vi "Intake_Hopper_Pneumatic_Safety_Interlocks.vi"(5 "extend delay(ms)":u32=1000, 7 "retract delay(ms)":u32=1000, 9 "Hopper Input":T1=enum."Reverse", 10 "Intake Input":T1=enum."Reverse") -> (1 "Hopper Output":T1=enum."Reverse", 2 "Intake Output":T1=enum."Reverse")   [LabVIEW 2019]
uses:
  <vilib>/Rock Robotics/WPI/Solenoid/WPI_SolenoidValue.ctl
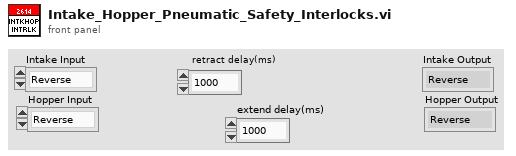
[diagram p1: front panel]
types:
  T1 = typedef "WPI_SolenoidValue.ctl" = enum16{"Off", "On", "Forward", "Reverse"}
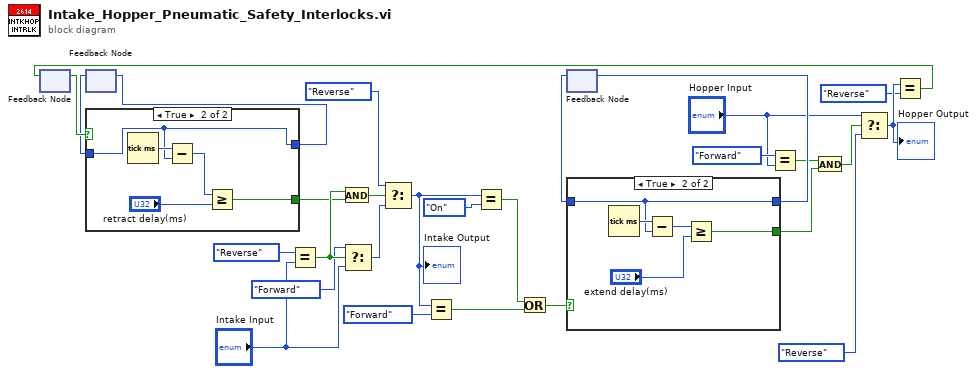
[diagram p0: block diagram]
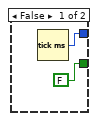
[diagram p2: hidden frame]
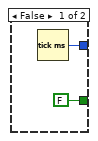
[diagram p3: hidden frame]
diagram:
  n1 = feedback #1() -> (w19:bool)  [unwired: 1 in]
  n2 = feedback #2() -> (w1:u32)  [unwired: 1 in]
  n3 = case shown="True" w19 {
    tunnel: [w29 w31] -> w2
    tunnel: [FALSE ("x .and. y?") w33] -> w20
    tunnel: w1 -> [_ w31]
    frame False {
      n4 = Tick Count (ms)() -> (millisecond timer value=w29:u32)
    }
    frame True {
      n5 = Tick Count (ms)() -> (millisecond timer value=w35:u32)
      n6 = Subtract(x=w35, y=w31) -> (x-y=w34:u32)
      n7 = Greater Or Equal?(x=w34, y="retract delay(ms)") -> (x >= y?=w33:bool)
    }
  }
  n8 = feedback-in #2(w2) -> ()
  n9 = Equal?(x=WPI_SolenoidValue."Reverse" ("y"), y="Intake Input") -> (x = y?=w21:bool)
  n10 = And(x=w21, y=w20) -> (x .and. y?=w22:bool)
  n11 = Select(t=WPI_SolenoidValue."Forward" ("y"), s=w21, f="Intake Input") -> (s? t:f=w16:T1)
  n12 = Select(t=WPI_SolenoidValue."Reverse" ("y"), s=w22, f=w16) -> (s? t:f=w4:T1)
  "Intake Output" <- w4
  n13 = Equal?(x=w4, y=WPI_SolenoidValue."Forward") -> (x = y?=w7:bool)
  n14 = Equal?(x=w4, y=WPI_SolenoidValue."On") -> (x = y?=w8:bool)
  n15 = Or(x=w8, y=w7) -> (x .or. y?=w23:bool)
  n16 = feedback #3() -> (w28:u32)  [unwired: 1 in]
  n17 = case shown="True" w23 {
    tunnel: [w37 w38] -> w27
    tunnel: [FALSE ("x .and. y?") w39] -> w25
    tunnel: w28 -> [_ w38]
    frame False {
      n18 = Tick Count (ms)() -> (millisecond timer value=w37:u32)
    }
    frame True {
      n19 = Tick Count (ms)() -> (millisecond timer value=w42:u32)
      n20 = Subtract(x=w42, y=w38) -> (x-y=w41:u32)
      n21 = Greater Or Equal?(x=w41, y="extend delay(ms)") -> (x >= y?=w39:bool)
    }
  }
  n22 = feedback-in #3(w27) -> ()
  n23 = Equal?(x=WPI_SolenoidValue."Forward" ("y"), y="Hopper Input") -> (x = y?=w26:bool)
  n24 = And(x=w26, y=w25) -> (x .and. y?=w24:bool)
  n25 = Select(t="Hopper Input", s=w24, f=WPI_SolenoidValue."Reverse" ("y")) -> (s? t:f=w11:T1)
  "Hopper Output" <- w11
  n26 = Equal?(x=w11, y=WPI_SolenoidValue."Reverse") -> (x = y?=w12:bool)
  n27 = feedback-in #1(w12) -> ()
